vi "Rename Broadcasts Cluster.vi"(8 "error in (no error)":errorcluster, 10 "Name":string, 11 "TargetRef in":refnum<vi>) -> (0 "error out":errorcluster)   [LabVIEW 2015, in "Generic Module Library.lvlib"]
uses:
  Generic Module Library.lvlib
panel:
  out "Text":string
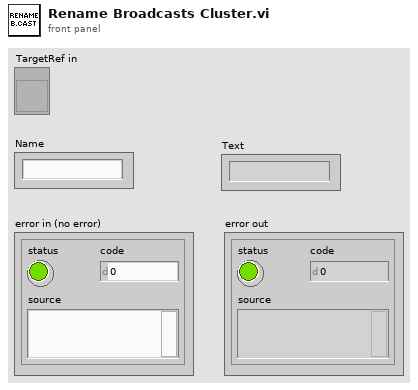
[diagram p1: front panel]
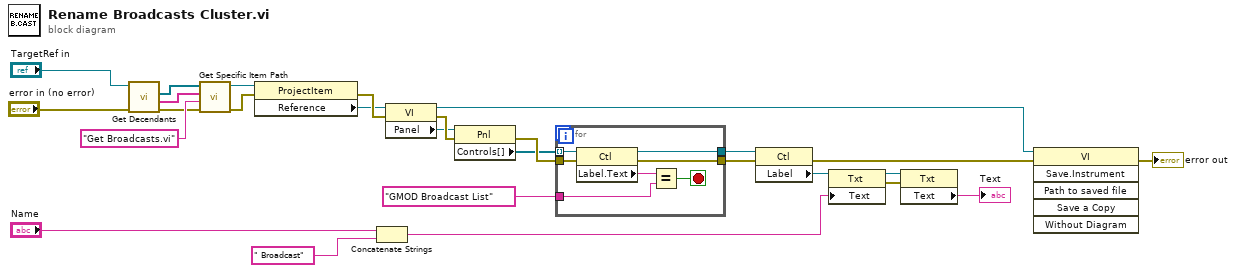
[diagram p0: block diagram]
diagram:
  n1 = call "Get Decendants.vi"("error in (no error)"="error in (no error)", "TargetRef in"="TargetRef in") -> ("error out"=w14:errorcluster, "Names"=w20:string[], "Decendant References"=w19:refnum<vi>[])  [unwired: 6 in, 1 out]
  n2 = call "Get Specific Item Path.vi"("error in (no error)"=w14, "Item to find"="Get Broadcasts.vi", "Names"=w20, "Decendant References"=w19) -> ("error out"=w21:errorcluster, "Item Reference"=w18:refnum<vi>)  [unwired: 4 in, 2 out]
  n3 = property class="ProjectItem"(reference=w18, error in=w21) -> (error out=w22:errorcluster, "Reference"=w13:refnum<vi>)  [unwired: 1 out]
  n4 = Concatenate Strings("Name", " Broadcast" ("string")) -> (w2:string)
  n5 = property class="VI"(reference=w13, error in=w22) -> (reference out=w3:refnum<vi>, error out=w23:errorcluster, "Panel"=w12:refnum<vi>)
  n6 = property class="Pnl"(reference=w12, error in=w23) -> (error out=w24:errorcluster, "Controls[]"=w11:refnum<vi>[])  [unwired: 1 out]
  n7 = for {
    tunnel: w11 -> [w34] mode=indexing
    tunnel: "GMOD Broadcast List" ("y") -> [w33]
    tunnel: [w31] -> w17
    tunnel: w24 -> [w30]
    tunnel: [w29] -> w25
    stop <- w32 stop-if-true
    n8 = property class="Ctl"(reference=w34, error in=w30) -> (reference out=w31:refnum<vi>, error out=w29:errorcluster, "Label.Text"=w28:string)
    n9 = Equal?(x=w28, y=w33) -> (x = y?=w32:bool)
  }
  n10 = property class="Ctl"(reference=w17, error in=w25) -> (error out=w27:errorcluster, "Label"=w10:refnum<vi>)  [unwired: 1 out]
  n11 = property class="Txt"(reference=w10, "Text"=w2) -> (reference out=w8:refnum<vi>, error out=w6:errorcluster)  [unwired: 1 in]
  n12 = property class="Txt"(reference=w8, error in=w6) -> ("Text"=→"Text":string)  [unwired: 2 out]
  n13 = invoke class="VI" method="Save.Instrument"(reference=w3, error in=w27) -> (error out=→"error out":errorcluster)  [unwired: 4 in, 5 out]
